vi "test_MultipleSessionsReserved_CallCreateSession_NothingAddedToCollectionMap.vi"(8 "error in":errorcluster) -> (0 "error out":errorcluster, 2 "result":string, 3 "pass":bool)   [LabVIEW 2020, in "MeasurementServerTests.lvlib"]
uses:
  MeasurementServerTests.lvlib
  Runtime/MeasurementLink Session Management/Session Reservation/Connection with Session.ctl
  Runtime/MeasurementLink Session Management/Session Reservation/Connection.ctl
  1a7c149c-48bc-4238-8756-811e337da54d.vi
  a956f7ee-c7e9-4639-884c-f4265dae6ecf.vi
  5728b933-7d39-4da4-b754-5b48616fa0f3.vi
  Helpers/Fake Instrument/Fake Instrument.lvclass
  C:/dev/measurementlink-labview/Source/Runtime/MeasurementLink Instrument/IInstrument/IInstrument.lvclass
  Runtime/MeasurementLink Session Management/Session Reservation/Create Sessions Dispatcher.vi
  Runtime/MeasurementLink Session Management/Session Reservation/Get Connections Dispatcher.vi
  Runtime/MeasurementLink Session Management/Session Reservation/Session Reservation.lvclass
  Runtime/MeasurementLink Measurement Server/Helpers/Error Strings Global Internal.vi
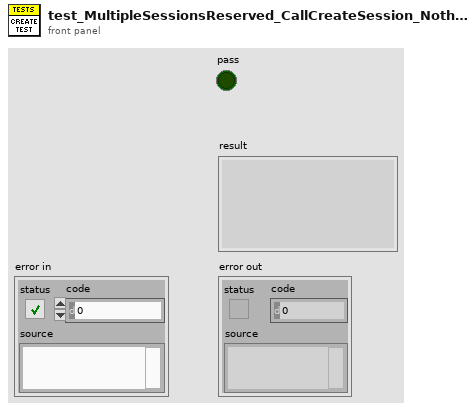
[diagram p1: front panel]
types:
  T1 = typedef "MeasurementLink Session Management.lvlib/Session Reservation.lvclass/Connection with Session.ctl" = cluster{"connection":T2, "session":variant}
  T2 = typedef "MeasurementLink Session Management.lvlib/Session Reservation.lvclass/Connection.ctl" = cluster{"pin or relay name":string, "site":i32, "instrument type id":string, "channel":string}
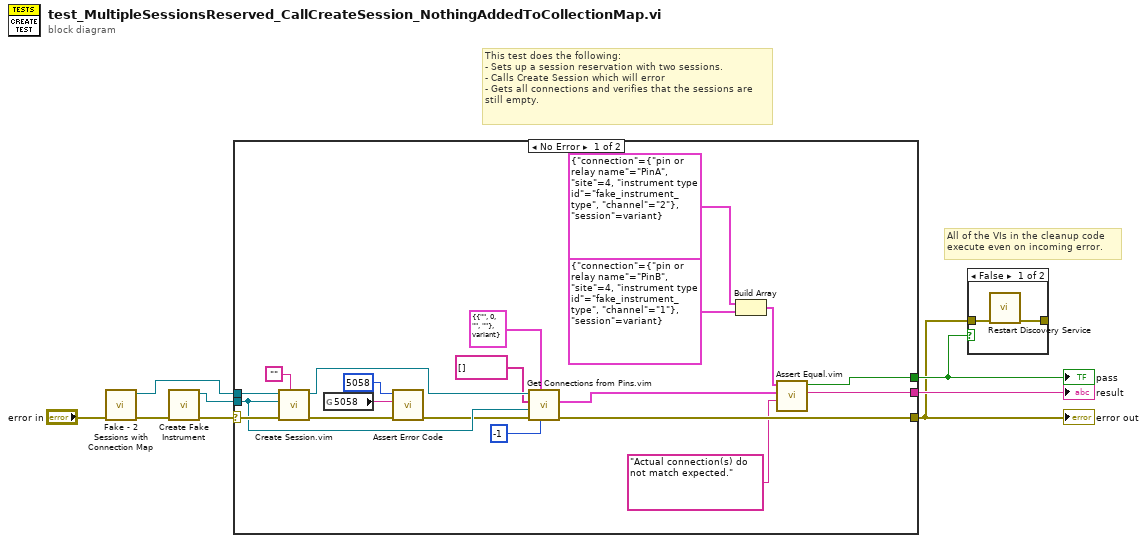
[diagram p0: block diagram]
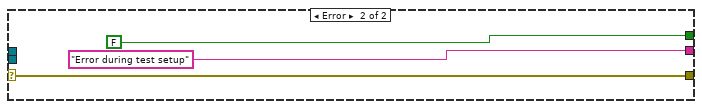
[diagram p2: hidden frame]
diagram:
  # "All of the VIs in the cleanup code\nexecute even on incoming error."
  # "This test does the following:\n- Sets up a session reservation with two sessions.\n- Calls Create Session which will error \n- Gets all connections and verifies that the sessions are\nstill empty."
  n1 = call "Fake - 2 Sessions with Connection Map.vi"("error in"="error in") -> ("error out"=w2:errorcluster, "session reservation out"=w1:refnum<class "Session Reservation.lvclass">)  [unwired: 9 in]
  n2 = call "Create Fake Instrument.vi"("error in"=w2) -> ("error out"=w5:errorcluster, "fake instrument out"=w4:refnum<class "Fake Instrument.lvclass">)  [unwired: 9 in]
  n3 = case shown="No Error" w5 {
    selector: w5 -> [w27 w29]
    tunnel: [w20 w29] -> w6
    tunnel: [w13 FALSE] -> w7
    tunnel: [w14 "Error during test setup" ("f")] -> w8
    tunnel: w4 -> [w23 _]
    tunnel: w1 -> [w28 _]
    frame No Error {
      n4 = call "Create Session.vim"("session type"="", "error in"=w27, "instrument"=w23, "session reservation in"=w28) -> ("error out"=w12:errorcluster, "session reservation out"=w25:refnum<class "Session Reservation.lvclass">)  [unwired: 4 in, 2 out]
      n5 = global read "Error Strings Global Internal.vi" "5058"() -> (w10:string)
      n6 = call "Assert Error Code.vi"("error in"=w12, "expected error description"=w10, "expected error code"=5058) -> ("error out"=w11:errorcluster)  [unwired: 6 in, 2 out]
      n7 = call "Get Connections from Pins.vim"("site"=-1, "connection type"=T1 {"connection"={"pin or relay name"="", "site"=0, "instrument type id"="", "channel"=""}, "session"=variant}, "error in"=w11, "instrument"=w23, "pin or relay names"=string[] [], "session reservation in"=w25) -> ("error out"=w20:errorcluster, "connections"=w19:T1[])  [unwired: 3 in, 1 out]
      n8 = Build Array(T1 {"connection"={"pin or relay name"="PinA", "site"=4, "instrument type id"="fake_instrument_type", "channel"="2"}, "session"=variant} ("connection out"), T1 {"connection"={"pin or relay name"="PinB", "site"=4, "instrument type id"="fake_instrument_type", "channel"="1"}, "session"=variant} ("connection out")) -> (w18:T1[])
      n9 = call "Assert Equal.vim"("failure message"="Actual connection(s) do not match expected.", "actual value"=w19, "expected value"=w18) -> ("message"=w14:string, "equal?"=w13:bool)  [unwired: 7 in]
    }
    frame Error {
    }
  }
  "error out" <- w6
  "pass" <- w7
  "result" <- w8
  n10 = case shown="False" w7 {
    tunnel: w6 -> [w33 _]
    tunnel: [w32 _] -> _
    frame False {
      n11 = call "Restart Discovery Service.vi"("error in"=w33) -> ("error out"=w32:errorcluster)  [unwired: 10 in]
    }
    frame True {
    }
  }
